vi "DataBuffer(SubVI).vi"(2 "Bits":dbl[](array[numeric]), 4 "Buffer":dbl[](array[numeric])) -> (0 "Data":dbl[](array[numeric]))   [LabVIEW 2017]
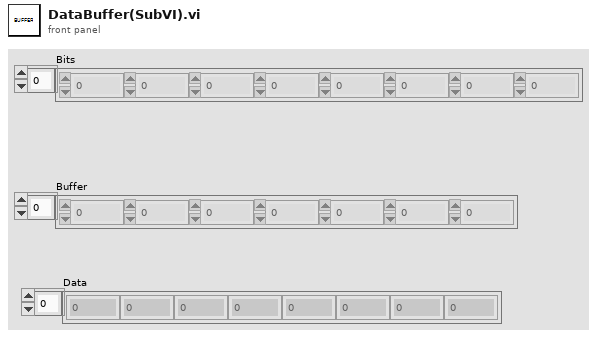
[diagram p1: front panel]
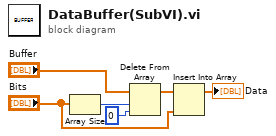
[diagram p0: block diagram]
diagram:
  n1 = Array Size(array="Bits") -> (size(s)=w6:i32)
  n2 = Delete From Array(array="Buffer", length=w6, index=0 ("비활성화된 인덱스 (열)")) -> (array with subset deleted=w4:dbl[])  [unwired: 1 out]
  n3 = Insert Into Array(array=w4, new element="Bits") -> (→"Data":dbl[])  [unwired: 1 in]
